vi "sub_identity-matrix.vi"(11 "STATE_SIZE":i32) -> (3 "identity":dbl[][](array[numeric]))   [LabVIEW 2019]
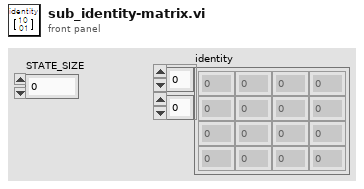
[diagram p1: front panel]
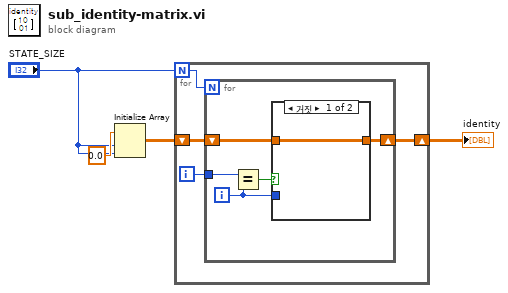
[diagram p0: block diagram]
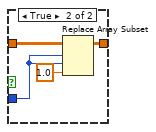
[diagram p2: hidden frame]
diagram:
  n1 = Initialize Array(0.0 ("원소"), "STATE_SIZE", "STATE_SIZE") -> (w4:dbl[][])
  n2 = for {
    N: "STATE_SIZE" -> [w8]
    shift-right: [w5] -> w1
    shift-left: w4 -> [w6]
    i -> [w7]
    n3 = for {
      N: w8 -> [_]
      tunnel: w7 -> [w13]
      shift-right: [w11] -> w5
      shift-left: w6 -> [w12]
      i -> [w10]
      n4 = Equal?(x=w13, y=w10) -> (x = y?=w9:bool)
      n5 = case shown="거짓" w9 {
        tunnel: w12 -> [w14 w18]
        tunnel: [w14 w17] -> w11
        tunnel: w10 -> [_ w16]
        frame False {
        }
        frame True {
          n6 = Replace Array Subset(array=w18, new element=1.0 ("새 원소/부분배열"), index (row)=w16, index (col)=w16) -> (w17:dbl[][])
        }
      }
    }
  }
  "identity" <- w1
